vi "GetSensorNames.vi"(11 "read buffer":string) -> (3 "sensors names":string[](array[string]))   [LabVIEW 2018]
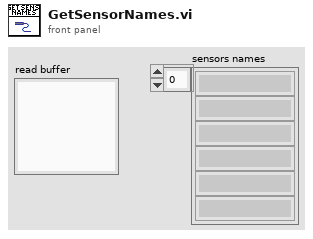
[diagram p1: front panel]
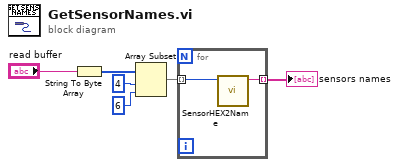
[diagram p0: block diagram]
diagram:
  n1 = String To Byte Array(string="read buffer") -> (unsigned byte array=w6:u8[])
  n2 = Array Subset(array=w6, index=4, length=6) -> (w3:u8[])
  n3 = for {
    tunnel: w3 -> [w8] mode=indexing
    tunnel: [w7] -> w4 mode=indexing
    n4 = call "SensorHEX2Name.vi"("Sensor HEX"=w8) -> ("Sensor name"=w7:string)  [unwired: 10 in]
  }
  "sensors names" <- w4
